vi "6502 Clock Gen And EEPROM Simulator.vi"() -> ()   [LabVIEW 2021]
uses:
  IO/IO.lvclass/IO.ctl
  EEPROM/EEPROM.lvclass/EEPROM.ctl
  IO/IO.lvclass
  EEPROM/EEPROM.lvclass
panel:
  out "Clock Frequency [Hz]":dbl format="%.3p"
  out "EEPROM":u8[](array[numeric]) format="%.0x"
  out "R/W":bool
  out "Data":u8 format="%04x"
  out "Data":bool[](array[boolean])
  out "CLK":bool
  in  "Single Step":bool
  in  "Free Running":bool
  in  "Clock Half Period [ms]":u32=1000
  out "Address":u16 format="%04x"
  out "Address":bool[](array[boolean])
  out "Address":u16(graph)
  # "Clock rising edge: setup data\n\nClock falling edge: sample data"
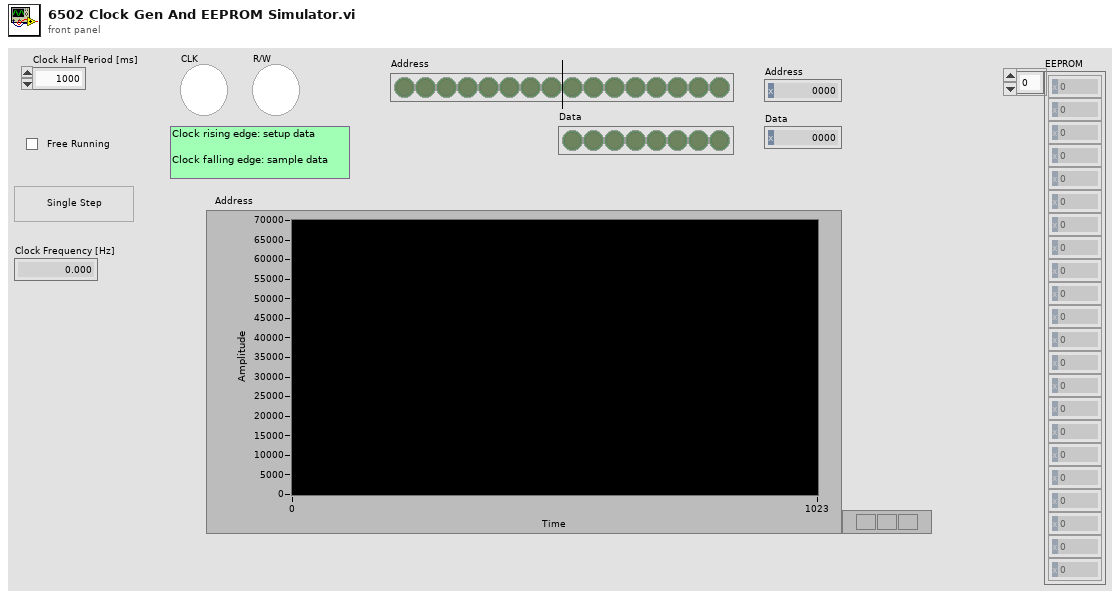
[diagram p1: front panel]
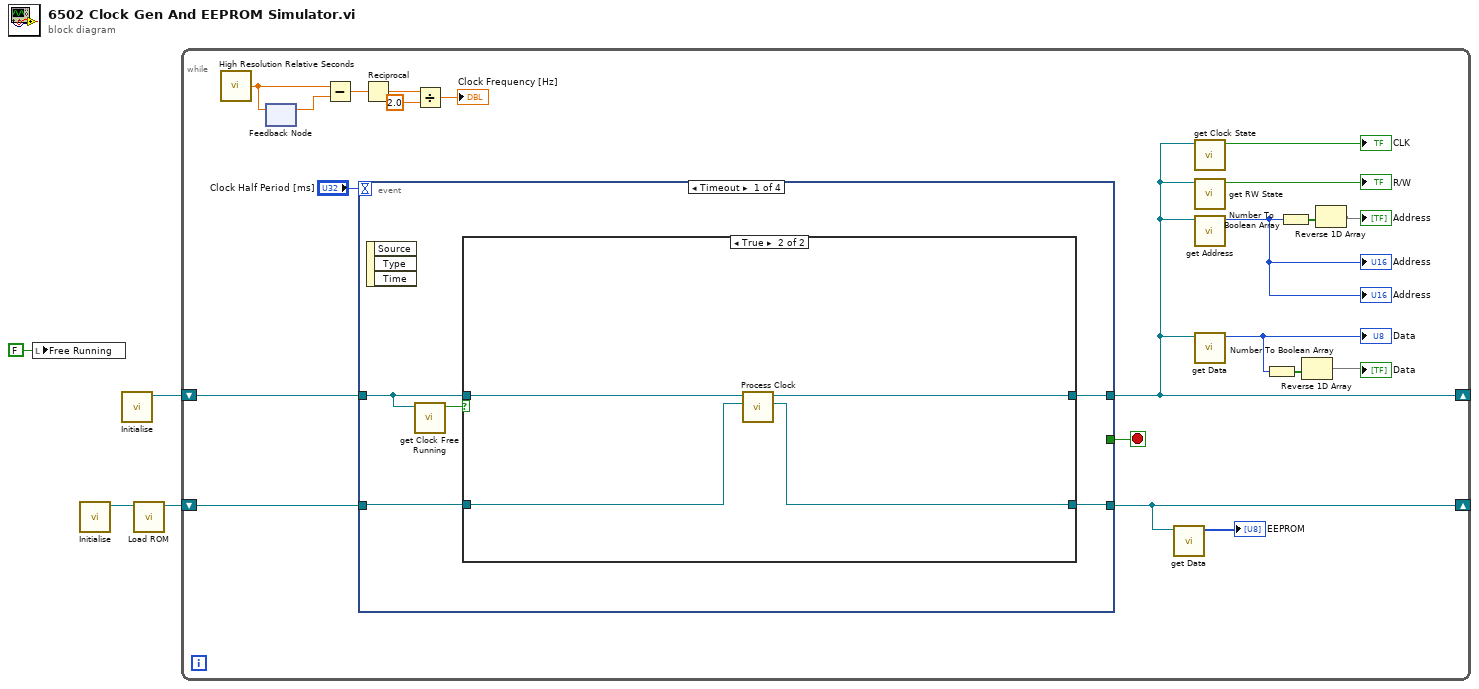
[diagram p0: block diagram]
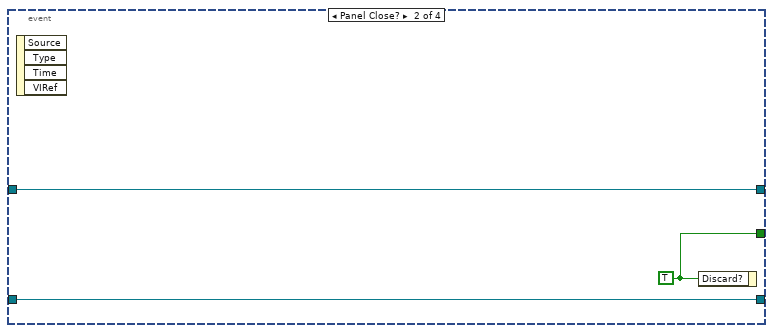
[diagram p3: hidden frame]
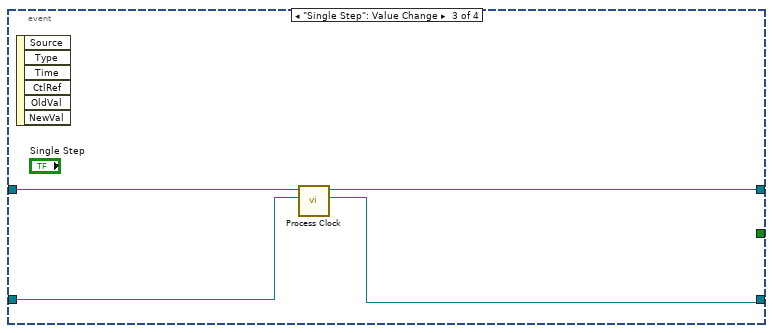
[diagram p4: hidden frame]
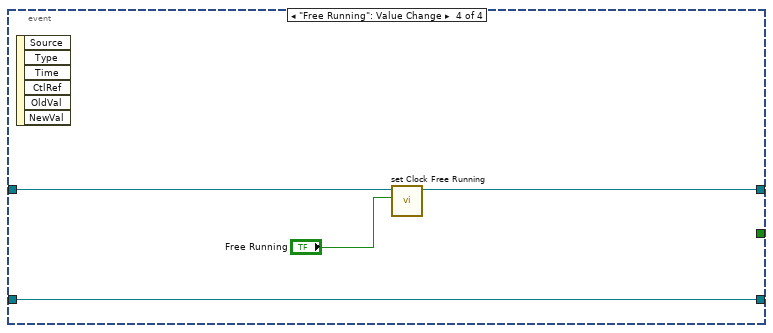
[diagram p5: hidden frame]
diagram:
  n1 = local write "Free Running"(FALSE ("Free Running")) -> ()
  n2 = call "Initialise.vi"() -> ("EEPROM out"=w2:refnum<class "EEPROM.lvclass">)  [unwired: 11 in]
  n3 = call "Initialise.vi"() -> ("Clock Generator"=w4:refnum<class "IO.lvclass">)  [unwired: 10 in, 1 out]
  n4 = call "Load ROM.vi"("EEPROM in"=w2) -> ("EEPROM out"=w1:refnum<class "EEPROM.lvclass">)  [unwired: 9 in, 1 out]
  n5 = while {
    shift-right: [w12] -> _
    shift-left: w1 -> [w23]
    shift-right: [w16] -> _
    shift-left: w4 -> [w22]
    stop <- w24 stop-if-true
    n6 = call <vilib>:"High Resolution Relative Seconds.vi"() -> ("relative seconds"=w10:dbl)
    n7 = feedback-in #1(w10) -> ()
    n8 = feedback #1() -> (w9:dbl)  [unwired: 1 in]
    n9 = Subtract(x=w10, y=w9) -> (x-y=w8:dbl)
    n10 = event shown="[0] Timeout" {
      selector: _ -> [_ _ _ _]
      dyn-events: _ -> [_ _ _ _]
      timeout: "Clock Half Period [ms]" -> [_ _ _ _]
      tunnel: [_ w39 _ _] -> w24
      tunnel: w23 -> [w29 w37 w41 w44]
      tunnel: [w30 w37 w40 w44] -> w12
      tunnel: w22 -> [w27 w38 w43 w47]
      tunnel: [w28 w38 w42 w46] -> w16
      event Timeout {
        n11 = event-data() -> ()  [unwired: 1 in, 3 out]
        n12 = call "get Clock Free Running.vi"("Clock Generator in"=w27) -> ("Free Running"=w26:bool)  [unwired: 10 in]
        n13 = case shown="True" w26 {
          tunnel: [w32 w36] -> w30
          tunnel: w29 -> [w32 w35]
          tunnel: w27 -> [w31 w34]
          tunnel: [w31 w33] -> w28
          frame False {
          }
          frame True {
            n14 = call "Process Clock.vi"("EEPROM in"=w35, "IO in"=w34) -> ("EEPROM out"=w36:refnum<class "EEPROM.lvclass">, "IO out"=w33:refnum<class "IO.lvclass">)  [unwired: 8 in]
          }
        }
      }
      event Panel Close? {
        w39 = TRUE ("Discard?")
        n15 = event-data() -> ()  [unwired: 1 in, 4 out]
        n16 = event-data("Discard?"=w39) -> ()  [unwired: 1 in, 1 out]
      }
      event "Single Step": Value Change {
        n17 = event-data() -> ()  [unwired: 1 in, 6 out]
        n18 = call "Process Clock.vi"("EEPROM in"=w41, "IO in"=w43) -> ("EEPROM out"=w40:refnum<class "EEPROM.lvclass">, "IO out"=w42:refnum<class "IO.lvclass">)  [unwired: 8 in]
      }
      event "Free Running": Value Change {
        n19 = event-data() -> ()  [unwired: 1 in, 6 out]
        n20 = call "set Clock Free Running.vi"("Free Running"="Free Running", "Clock Generator in"=w47) -> ("Clock Generator out"=w46:refnum<class "IO.lvclass">)  [unwired: 9 in]
      }
    }
    n21 = Reciprocal(x=w8) -> (1/x=w7:dbl)
    n22 = Divide(x=w7, y=2.0) -> (x/y=→"Clock Frequency [Hz]":dbl)
    n23 = call "get Data.vi"("EEPROM in"=w12) -> ("Data"=→"EEPROM":u8[])  [unwired: 10 in]
    n24 = call "get Clock State.vi"("Clock Generator in"=w16) -> ("Current State"=→"CLK":bool)  [unwired: 10 in]
    n25 = call "get RW State.vi"("IO in"=w16) -> ("R/W State"=→"R/W":bool)  [unwired: 10 in]
    n26 = call "get Address.vi"("IO in"=w16) -> ("Address"=w17:u16)  [unwired: 10 in]
    "Address" <- w17
    "Address" <- w17
    n27 = call "get Data.vi"("IO in"=w16) -> ("Data"=w14:u8)  [unwired: 10 in]
    "Data" <- w14
    n28 = Number To Boolean Array(number=w14) -> (Boolean array=w15:bool[])
    n29 = Number To Boolean Array(number=w17) -> (Boolean array=w20:bool[])
    n30 = Reverse 1D Array(array=w15) -> (reversed array=→"Data":bool[])
    n31 = Reverse 1D Array(array=w20) -> (reversed array=→"Address":bool[])
  }
